vi "Get XY Graph Y Mapping.vi"(8 "error in (no error)":errorcluster, 11 "graph_utilities in":refnum<class "graph_utilities.lvclass">) -> (0 "error out":errorcluster, 2 "Y Scale Mapping":T1 items=["Linear", "Logarithmic"], 3 "graph_utilities out":refnum<class "graph_utilities.lvclass">)   [LabVIEW 2016, in "graph_utilities.lvclass"]
doc: "Get the Y Scale Mapping (linear or logarithmic)."
uses:
  graph_utilities.lvclass
  Typedefs/Scale Mapping  - Enum.ctl
  graph_utilities.lvclass/graph_utilities.ctl
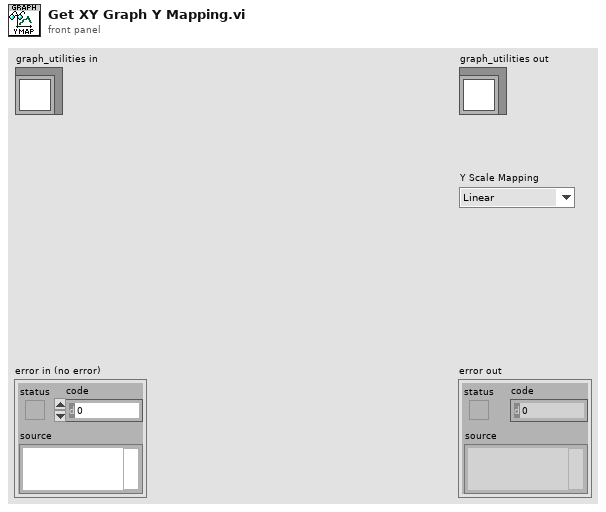
[diagram p1: front panel]
types:
  T1 = typedef "graph_utilities.lvclass/Scale Mapping  - Enum.ctl" = u16
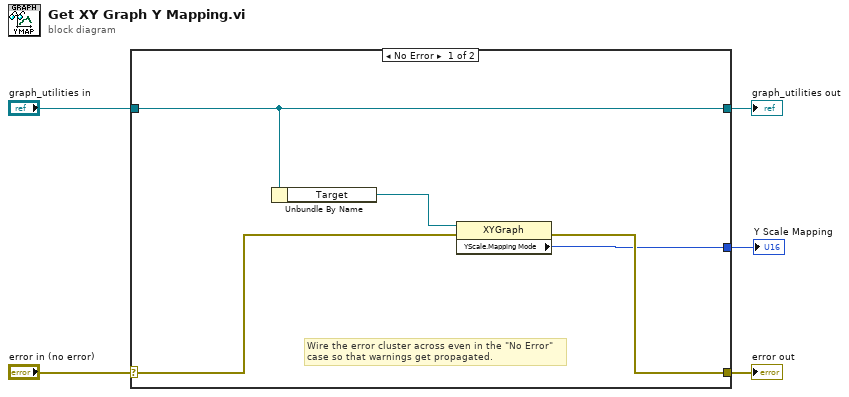
[diagram p0: block diagram]
diagram:
  n1 = case shown="No Error" "error in (no error)" {
    selector: "error in (no error)" -> [w8 w12]
    tunnel: [w7 w12] -> w4
    tunnel: [w10 w11] -> w2
    tunnel: "graph_utilities in" -> [w10 w11]
    tunnel: [w6 _] -> w1
    frame No Error {
      # "Wire the error cluster across even in the \"No Error\"\ncase so that warnings get propagated."
      n2 = Unbundle By Name(w10) -> ("Target"=w9:refnum<vi>)
      n3 = property on="Property Node" class="XYGraph"(reference=w9, error in=w8) -> (error out=w7:errorcluster, "YScale.Mapping Mode"=w6:u8)  [unwired: 1 out]
    }
    frame Error {
    }
  }
  "error out" <- w4
  "graph_utilities out" <- w2
  "Y Scale Mapping" <- w1
